vi "GraphFitting.vi"(8 "L_Threshold":dbl, 9 "R_Threshold":dbl, 10 "width":i32=15, 11 "signal":waveform(dbl)) -> (2 "출력 웨이브폼 2":waveform(dbl) caption="Org", 3 "출력 웨이브폼":waveform(dbl) caption="Fitted")   [LabVIEW 2012]
uses:
  <vilib>/addons/Wavelet Analysis/application.llb/WA Multiscale Peak Detection (Waveform).vi
  <vilib>/addons/_Advanced Signal Processing/NI_AdvSigProcWA.lvlib
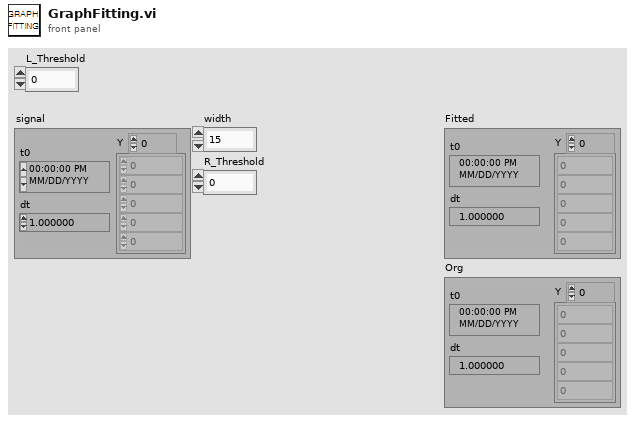
[diagram p1: front panel]
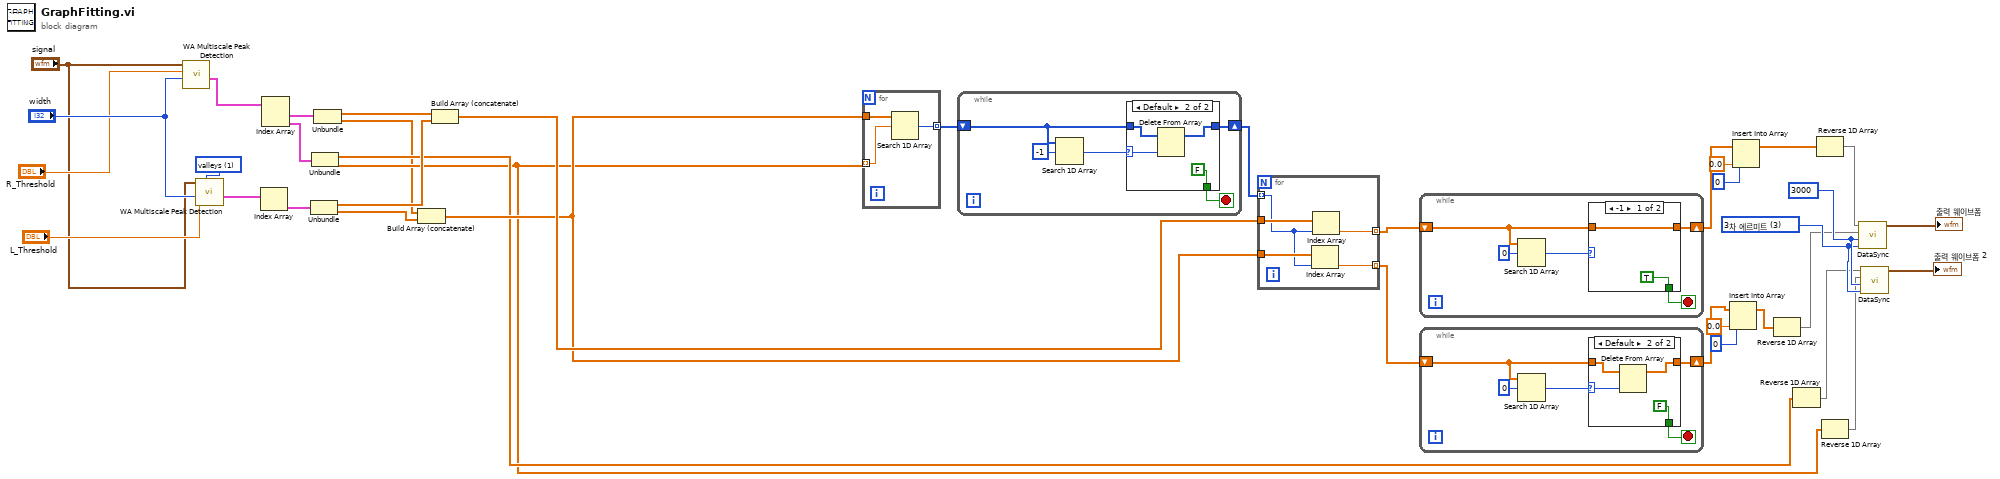
[diagram p0: block diagram]
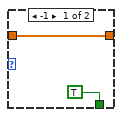
[diagram p2: hidden frame]
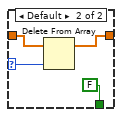
[diagram p3: hidden frame]
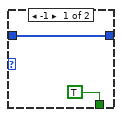
[diagram p4: hidden frame]
diagram:
  w23 = 3 items=["최근접", "선형", "스플라인", "3차 에르미트", "라그랑지"] ("method")
  w24 = 3000 ("samples")
  w38 = u16 1 items=["peaks", "valleys"] ("peaks/valleys")
  n1 = call-poly <vilib>:"WA Multiscale Peak Detection.vi"("width"="width", "threshold"="R_Threshold", "signal"="signal") -> ("peak plot"=w25:cluster{"Ramp Pattern":dbl[], "X":dbl[]}[])  [unwired: 4 in, 4 out]
  n2 = call-poly <vilib>:"WA Multiscale Peak Detection.vi"("peaks/valleys"=w38, "width"="width", "threshold"="L_Threshold", "signal"="signal") -> ("peak plot"=w37:cluster{"Ramp Pattern":dbl[], "X":dbl[]}[])  [unwired: 3 in, 4 out]
  n3 = Index Array(array=w37) -> (element=w26:cluster{"Ramp Pattern":dbl[], "X":dbl[]})  [unwired: 1 in]
  n4 = Index Array(array=w25) -> (element #1=w36:cluster{"Ramp Pattern":dbl[], "X":dbl[]}, element #2=w35:cluster{"Ramp Pattern":dbl[], "X":dbl[]})  [unwired: 2 in]
  n5 = Unbundle(w26) -> ("Ramp Pattern"=w34:dbl[], "X"=w33:dbl[])
  n6 = Unbundle(w35) -> ("Ramp Pattern"=w11:dbl[], "X"=w9:dbl[])
  n7 = Unbundle(w36) -> ("Ramp Pattern"=w1:dbl[], "X"=w4:dbl[])
  n8 = Build Array (concatenate)(w4, w33) -> (w31:dbl[])
  n9 = Build Array (concatenate)(w1, w34) -> (w32:dbl[])
  n10 = for {
    tunnel: w9 -> [w40] mode=indexing
    tunnel: w31 -> [w41]
    tunnel: [w39] -> w30 mode=indexing
    n11 = Search 1D Array(1D array=w41, element=w40) -> (index of element=w39:i32)  [unwired: 1 in]
  }
  n12 = while {
    shift-right: [w46] -> w29
    shift-left: w30 -> [w45]
    stop <- w43 stop-if-true
    n13 = Search 1D Array(1D array=w45, element=-1) -> (index of element=w44:i32)  [unwired: 1 in]
    n14 = case shown="Default" w44 {
      selector: w44 -> [_ w50]
      tunnel: w45 -> [w48 w52]
      tunnel: [w48 w51] -> w46
      tunnel: [TRUE FALSE] -> w43
      frame -1 {
      }
      frame Default {
        n15 = Delete From Array(array=w52, index=w50) -> (array with subset deleted=w51:i32[])  [unwired: 1 in, 1 out]
      }
    }
  }
  n16 = for {
    tunnel: w29 -> [w55] mode=indexing
    tunnel: w32 -> [w57]
    tunnel: w31 -> [w56]
    tunnel: [w54] -> w28 mode=indexing
    tunnel: [w53] -> w27 mode=indexing
    n17 = Index Array(array=w56, index=w55) -> (element=w53:dbl)
    n18 = Index Array(array=w57, index=w55) -> (element=w54:dbl)
  }
  n19 = while {
    shift-right: [w62] -> w21
    shift-left: w28 -> [w61]
    stop <- w59 stop-if-true
    n20 = Search 1D Array(1D array=w61, element=0) -> (index of element=w60:i32)  [unwired: 1 in]
    n21 = case shown="-1" w60 {
      selector: w60 -> [_ w66]
      tunnel: w61 -> [w64 w68]
      tunnel: [w64 w67] -> w62
      tunnel: [TRUE FALSE] -> w59
      frame -1 {
      }
      frame Default {
        n22 = Delete From Array(array=w68, index=w66) -> (array with subset deleted=w67:dbl[])  [unwired: 1 in, 1 out]
      }
    }
  }
  n23 = while {
    shift-right: [w73] -> w19
    shift-left: w27 -> [w72]
    stop <- w70 stop-if-true
    n24 = Search 1D Array(1D array=w72, element=0) -> (index of element=w71:i32)  [unwired: 1 in]
    n25 = case shown="Default" w71 {
      selector: w71 -> [_ w77]
      tunnel: w72 -> [w75 w79]
      tunnel: [w75 w78] -> w73
      tunnel: [TRUE FALSE] -> w70
      frame -1 {
      }
      frame Default {
        n26 = Delete From Array(array=w79, index=w77) -> (array with subset deleted=w78:dbl[])  [unwired: 1 in, 1 out]
      }
    }
  }
  n27 = Insert Into Array(array=w19, index=0, new element=0.0 ("new element/subarray")) -> (w13:dbl[])
  n28 = Insert Into Array(array=w21, index=0, new element=0.0 ("new element/subarray")) -> (w15:dbl[])
  n29 = Reverse 1D Array(array=w13) -> (reversed array=w12:dbl[])
  n30 = Reverse 1D Array(array=w11) -> (reversed array=w10:dbl[])
  n31 = Reverse 1D Array(array=w15) -> (reversed array=w14:dbl[])
  n32 = Reverse 1D Array(array=w9) -> (reversed array=w8:dbl[])
  n33 = call "DataSync.vi"("method"=w23, "samples"=w24, "Y"=w12, "X"=w14) -> ("출력 웨이브폼"=→"출력 웨이브폼":waveform(dbl))  [unwired: 5 in, 2 out]
  n34 = call "DataSync.vi"("method"=w23, "samples"=w24, "Y"=w8, "X"=w10) -> ("출력 웨이브폼"=→"출력 웨이브폼 2":waveform(dbl))  [unwired: 5 in, 2 out]
